vi "nanomsg_get_attrs.vi"(3 "ref array":refnum<vi>[](array[refnum])) -> (0 "size":i32, 1 "attrs":i32[](array[numeric]))   [LabVIEW 2014]
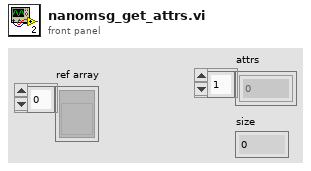
[diagram p1: front panel]
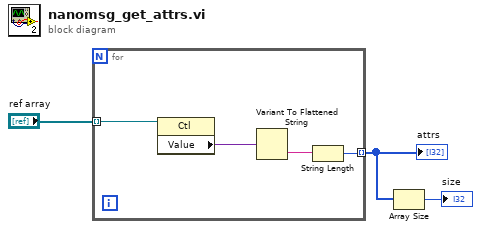
[diagram p0: block diagram]
diagram:
  n1 = for {
    tunnel: "ref array" -> [w7] mode=indexing
    tunnel: [w4] -> w2 mode=indexing
    n2 = property class="Ctl"(reference=w7) -> ("Value"=w6:variant)  [unwired: 1 in, 2 out]
    n3 = Variant To Flattened String(Variant=w6) -> (data string=w5:string)  [unwired: 1 out]
    n4 = String Length(string=w5) -> (length=w4:i32)
  }
  "attrs" <- w2
  n5 = Array Size(array=w2) -> (size(s)=→"size":i32)
